vi "Flush Queue.vi"(8 "error in (no error)":errorcluster, 9 "Option (Low Priority As Default)":enum16{"All", "High Priority", "Low Priority"}(ring)=enum."Low Priority", 11 "Priority Queue In":T5) -> (0 "error out":errorcluster, 1 "Remaining Elements (Low)":T1[](array[typedef]), 2 "Remaining Elements (Hight)":T2[](array[typedef]), 3 "Priority Queue Out":T5)   [LabVIEW 2017, in "Communicable State Machine.lvlib"]
uses:
  Communicable State Machine.lvlib
  Priority Queue.ctl
  Typedef/_Cross CSM State Data.ctl
  Typedef/_CSM_MSG_TYPE.ctl
  Typedef/_Cross CSM State Response.ctl
  Typedef/_CSM_Response Source Message.ctl
  def-Data(LowPRI-Q).ctl
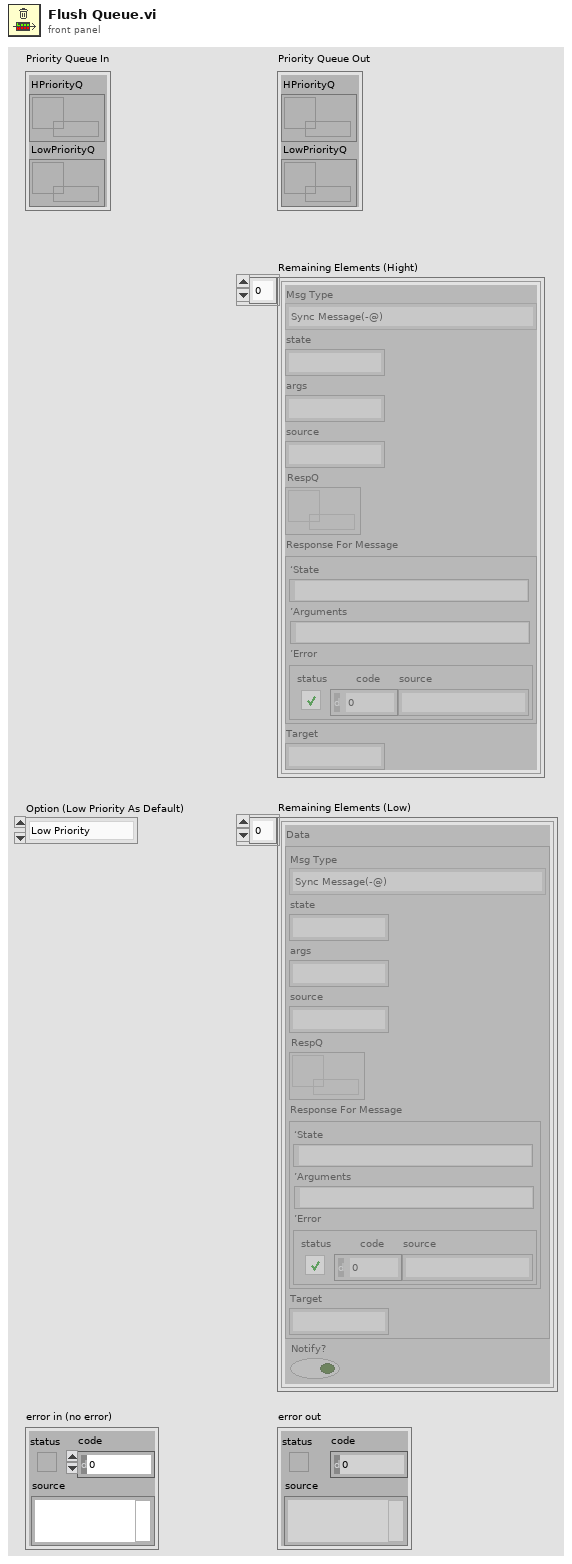
[diagram p1: front panel]
types:
  T1 = typedef "Communicable State Machine.lvlib/def-Data(LowPRI-Q).ctl" = cluster{"Data":T2, "Notify?":bool}
  T2 = typedef "Communicable State Machine.lvlib/_Cross CSM State Data.ctl" = cluster{"Msg Type":T3, "state":string, "args":string, "source":string, "RespQ":refnum<queue>, "Response For Message":T4, "Target":string}
  T3 = typedef "Communicable State Machine.lvlib/_CSM_MSG_TYPE.ctl" = enum16{"Sync Message(-@)", "Async Message(->)", "Async without Response(->|)", "Async Response", "Broadcast(-><all>)", "Broadcast(-><status>)", "Broadcast(-><interrupt>)", "Append to JKISM States", "Append to JKISM States(High Priority)", "Broadcast(-><state>)"}
  T4 = typedef "Communicable State Machine.lvlib/_CSM_Response Source Message.ctl" = cluster{"‘State":string, "’Arguments":string, "’Error":errorcluster}
  T5 = typedef "Communicable State Machine.lvlib/Priority Queue.ctl" = cluster{"HPriorityQ":refnum<queue>, "LowPriorityQ":refnum<queue>}
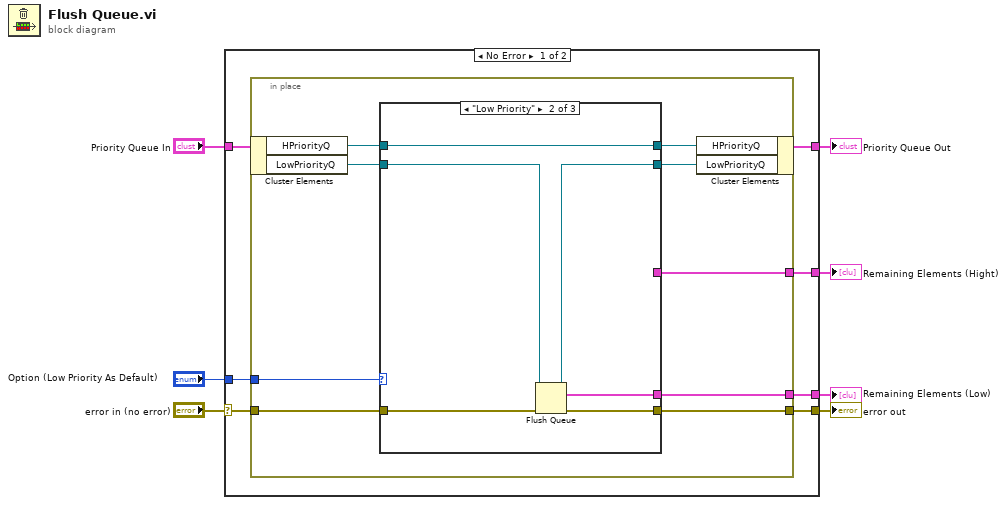
[diagram p0: block diagram]
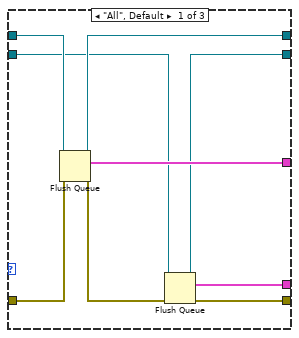
[diagram p2: hidden frame]
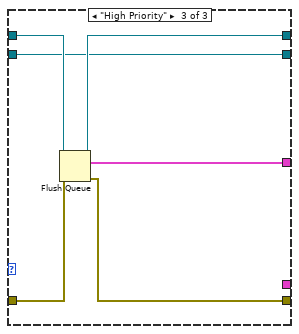
[diagram p3: hidden frame]
diagram:
  n1 = case shown="No Error" "error in (no error)" {
    selector: "error in (no error)" -> [w14 w46]
    tunnel: [w13 w46] -> w6
    tunnel: [w12 _] -> w5
    tunnel: [w11 _] -> w4
    tunnel: "Priority Queue In" -> [w10 w45]
    tunnel: [w9 w45] -> w2
    tunnel: "Option (Low Priority As Default)" -> [w8 _]
    frame No Error {
      n2 = in-place {
        in-place-border: w14 -> [w23]
        in-place-border: [w22] -> w13
        in-place-border: [w21] -> w12
        in-place-border: [w20] -> w11
        in-place-border: w8 -> [w15]
        n3 = in-place-cluster #1(w10) -> ("HPriorityQ"=w18:refnum<queue>, "LowPriorityQ"=w17:refnum<queue>)
        n4 = case shown="\"Low Priority\"" w15 {
          tunnel: w23 -> [w32 w38 w44]
          tunnel: [w30 w37 w43] -> w22
          tunnel: [w29 _ w42] -> w21
          tunnel: [w28 w36 _] -> w20
          tunnel: [w27 w35 w41] -> w19
          tunnel: w18 -> [w26 w35 w40]
          tunnel: w17 -> [w25 w34 w39]
          tunnel: [w24 w33 w39] -> w16
          frame "All", Default {
            n5 = Flush Queue(queue=w26, error in (no error)=w32) -> (queue out=w27:refnum<queue>, remaining elements=w29:T2[], error out=w31:errorcluster)
            n6 = Flush Queue(queue=w25, error in (no error)=w31) -> (queue out=w24:refnum<queue>, remaining elements=w28:T1[], error out=w30:errorcluster)
          }
          frame "Low Priority" {
            n7 = Flush Queue(queue=w34, error in (no error)=w38) -> (queue out=w33:refnum<queue>, remaining elements=w36:T1[], error out=w37:errorcluster)
          }
          frame "High Priority" {
            n8 = Flush Queue(queue=w40, error in (no error)=w44) -> (queue out=w41:refnum<queue>, remaining elements=w42:T2[], error out=w43:errorcluster)
          }
        }
        n9 = in-place-cluster #1("HPriorityQ"=w19, "LowPriorityQ"=w16) -> (w9:T5)
      }
    }
    frame Error {
    }
  }
  "error out" <- w6
  "Priority Queue Out" <- w2
  "Remaining Elements (Hight)" <- w5
  "Remaining Elements (Low)" <- w4
